vi "LOG Update LOG window.vi"(5 "String":string, 7 "replace":bool, 8 "error in (no error)":errorcluster, 11 "strLOG in":refnum<vi>) -> (0 "error out":errorcluster, 3 "strLOG out":refnum<vi>)   [LabVIEW 2020, in "LOG.lvlib"]
uses:
  LOG.lvlib
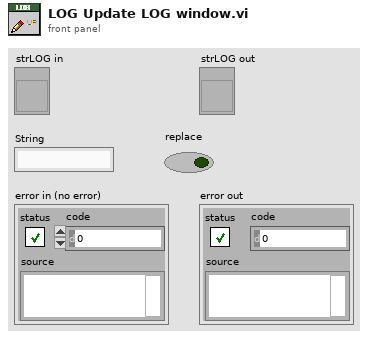
[diagram p1: front panel]
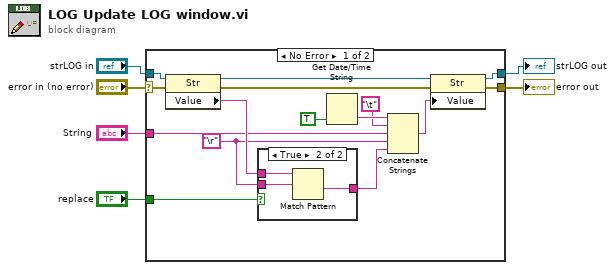
[diagram p0: block diagram]
diagram:
  n1 = case shown="No Error" "error in (no error)" {
    selector: "error in (no error)" -> [w9 w27]
    tunnel: [w15 w26] -> w6
    tunnel: "replace" -> [w12 _]
    tunnel: "strLOG in" -> [w10 w26]
    tunnel: [w8 w27] -> w2
    tunnel: "String" -> [w7 _]
    frame No Error {
      w13 = "\r"
      n2 = property class="Str"(reference=w10, error in=w9) -> (reference out=w19:refnum<vi>, error out=w21:errorcluster, "Value"=w14:string)
      n3 = case shown="True" w12 {
        tunnel: w14 -> [w22 w25]
        tunnel: w13 -> [_ w24]
        tunnel: [w22 w23] -> w11
        frame False {
        }
        frame True {
          n4 = Match Pattern(string=w25, regular expression=w24) -> (after substring=w23:string)  [unwired: 1 in, 3 out]
        }
      }
      n5 = Get Date/Time String(want seconds? (F)=TRUE) -> (time string=w17:string)  [unwired: 2 in, 1 out]
      n6 = Concatenate Strings(w17, "\t", w7, w13, w11) -> (w20:string)
      n7 = property class="Str"(reference=w19, error in=w21, "Value"=w20) -> (reference out=w15:refnum<vi>, error out=w8:errorcluster)
    }
    frame Error {
    }
  }
  "strLOG out" <- w6
  "error out" <- w2
